vi "mainvi.vi"() -> ()   [LabVIEW 2019]
panel:
  out "A+b":bool[][](array[boolean])
  out "A+B":dbl
  out "B":bool[](array[boolean])
  out "A":bool[](array[boolean])
  in  "B":dbl
  in  "A":dbl
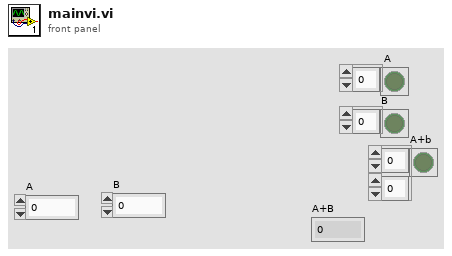
[diagram p1: front panel]
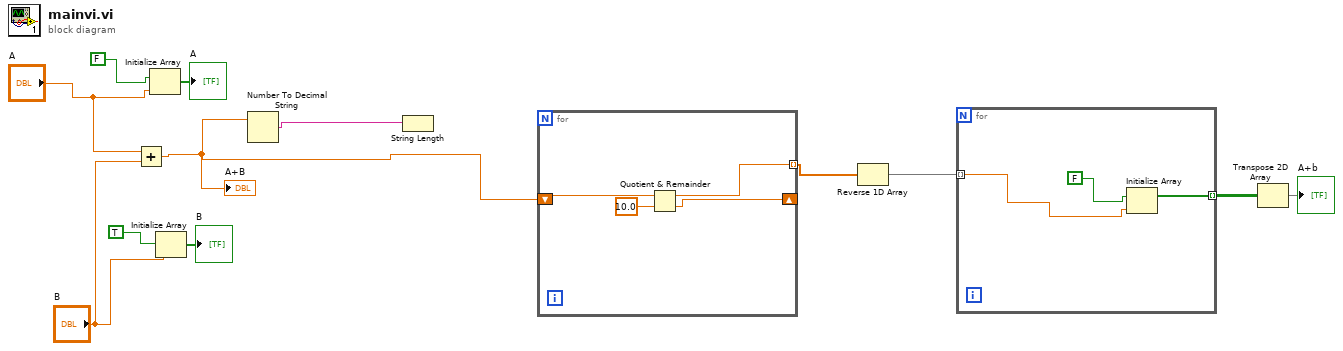
[diagram p0: block diagram]
diagram:
  n1 = Add(x="A", y="B") -> (x+y=w5:dbl)
  "A+B" <- w5
  n2 = Initialize Array(FALSE, "A") -> (→"A":bool[])
  n3 = Initialize Array(TRUE, "B") -> (→"B":bool[])
  n4 = Number To Decimal String(number=w5) -> (decimal integer string=w6:string)  [unwired: 1 in]
  n5 = String Length(string=w6) -> ()  [unwired: 1 out]
  n6 = for {
    shift-right: [w16] -> _
    shift-left: w5 -> [w15]
    tunnel: [w13] -> w4 mode=indexing
    n7 = Quotient & Remainder(x=w15, y=10.0) -> (x-y*floor(x/y)=w13:dbl, floor(x/y)=w16:dbl)
  }
  n8 = Reverse 1D Array(array=w4) -> (reversed array=w3:dbl[])
  n9 = for {
    tunnel: w3 -> [w18] mode=indexing
    tunnel: [w17] -> w2 mode=indexing
    n10 = Initialize Array(FALSE, w18) -> (w17:bool[])
  }
  n11 = Transpose 2D Array(2D array=w2) -> (transposed array=→"A+b":bool[][])
